vi "40exportToBdd.vi"(6 "Dcir":dbl, 7 "dcirOK?":bool, 9 "Datain":T1, 10 "test OK?":bool, 11 "SN":string="0B5MEVA000CA1JC1M0000041") -> (0 "error out":errorcluster, 2 "PLC requet":string, 3 "chaîne concaténée":string)   [LabVIEW 2020]
uses:
  VarGLO/Global var.vi
panel:
  in  "errin":errorcluster
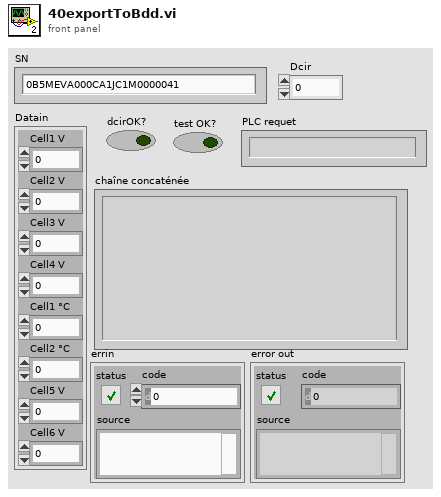
[diagram p1: front panel]
types:
  T1 = cluster{"Cell1 V":sgl, "Cell2 V":sgl, "Cell3 V":sgl, "Cell4 V":sgl, "Cell1 °C":sgl, "Cell2 °C":sgl, "Cell5 V":sgl, "Cell6 V":sgl}
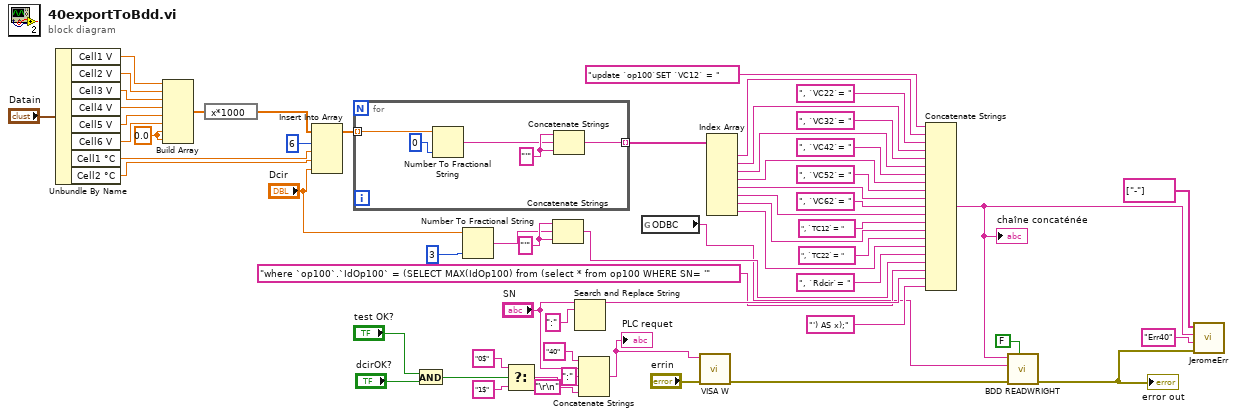
[diagram p0: block diagram]
diagram:
  w5 = "'" ("chaîne")
  w55 = sgl 0.0 ("element")
  n1 = Unbundle By Name("Datain") -> ("Cell1 V"=w48:sgl, "Cell2 V"=w49:sgl, "Cell3 V"=w50:sgl, "Cell4 V"=w51:sgl, "Cell5 V"=w52:sgl, "Cell6 V"=w53:sgl, "Cell1 °C"=w56:sgl, "Cell2 °C"=w57:sgl)
  n2 = Build Array(w48, w49, w50, w51, w52, w53, w55, w55) -> (w16:sgl[])
  n3 = expression code="x*1000"(w16) -> (w15:sgl[])
  n4 = Insert Into Array(array=w15, index=6 ("indice"), new element #1=w56, new element #2=w57, new element #3="Dcir") -> (w13:sgl[])
  n5 = for {
    tunnel: w13 -> [w65] mode=indexing
    tunnel: [w62] -> w22 mode=indexing
    w63 = "'" ("chaîne")
    n6 = Number To Fractional String ("Nombre en chaîne fractionnaire")(number=w65, precision (6)=i16 0 ("précision (6)")) -> (F-format string=w61:string)  [unwired: 2 in]
    n7 = Concatenate Strings(w63, w61, w63) -> (w62:string)
  }
  n8 = And(x="test OK?", y="dcirOK?") -> (x .and. y?=w40:bool)
  n9 = Number To Fractional String ("Nombre en chaîne fractionnaire")(number="Dcir", precision (6)=i16 3 ("précision (6)")) -> (F-format string=w4:string)  [unwired: 2 in]
  n10 = Select(t="0$" ("chaîne"), s=w40, f="1$" ("chaîne")) -> (s? t:f=w42:string)
  n11 = Concatenate Strings(w5, w4, w5) -> (w3:string)
  n12 = Search and Replace String ("Rechercher et remplacer une chaîne")(input string="SN", search string=":" ("chaîne recherchée")) -> (result string=w20:string)  [unwired: 6 in, 3 out]
  n13 = Concatenate Strings("40" ("chaîne"), "SN", ":" ("string"), w42, "\r\n") -> (w47:string)
  "PLC requet" <- w47
  n14 = global read "Global var.vi" "ODBC"() -> (w2:string)
  n15 = call "VISA W.vi"("errin"="errin", "Chaîne"=w47) -> ("errout"=w10:errorcluster)  [unwired: 9 in]
  n16 = Index Array(array=w22) -> (element #1=w23:string, element #2=w25:string, element #3=w27:string, element #4=w29:string, element #5=w31:string, element #6=w33:string, element #7=w34:string, element #8=w37:string)  [unwired: 8 in]
  n17 = Concatenate Strings("update `op100`SET `VC12` = " ("chaîne"), w23, ", `VC22`= " ("chaîne"), w25, ", `VC32`= " ("chaîne"), w27, ", `VC42`= " ("chaîne"), w29, ", `VC52`= " ("chaîne"), w31, ", `VC62`= " ("chaîne"), w33, ", `TC12`= " ("chaîne"), w34, ", `TC22`= " ("chaîne"), w37, ", `Rdcir`= " ("string"), w3, "where `op100`.`IdOp100` = (SELECT MAX(IdOp100) from (select * from op100 WHERE SN= '" ("chaîne"), w20, "') AS x);" ("chaîne")) -> (w8:string)
  "chaîne concaténée" <- w8
  n18 = call <userlib>:"BDD READWRIGHT.vi"("Read?"=FALSE, "errin"=w10, "DSN name"=w2, "Instruction"=w8) -> ("error out"=w9:errorcluster)  [unwired: 6 in, 1 out]
  "error out" <- w9
  n19 = call "JeromeErr.vi"("Errin"=w9, "CodeERR"="Err40", "RequetteSQL"=w8, "RetourSQL"=string[] ["-"]) -> ()  [unwired: 8 in]
